vi "Return Transfer Group.vi"(8 "error in (no error)":errorcluster, 10 "Transfer Group in":refnum<class "Transfer Group.lvclass">, 11 "Transceiver Thread in":refnum<class "Plugin Thread.lvclass">) -> (0 "error out":errorcluster, 3 "Transceiver Thread out":refnum<class "Plugin Thread.lvclass">)   [LabVIEW 2017, in "DSF Core.lvlib" / "Plugin Thread.lvclass"]
uses:
  Thread/Plugin/Plugin Thread.lvclass
  Transfer Group/Transfer Group.lvclass
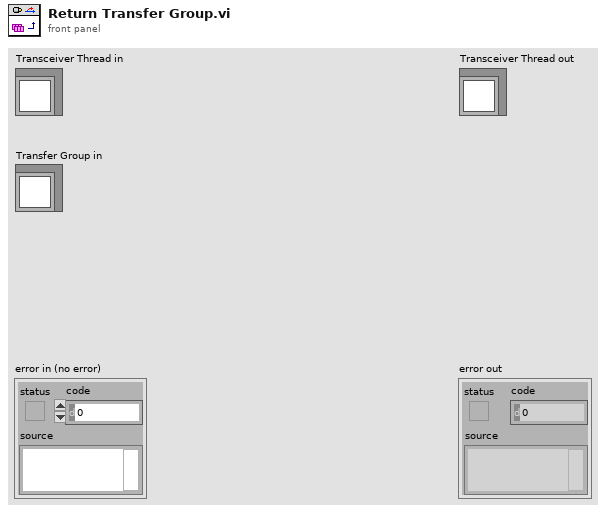
[diagram p1: front panel]
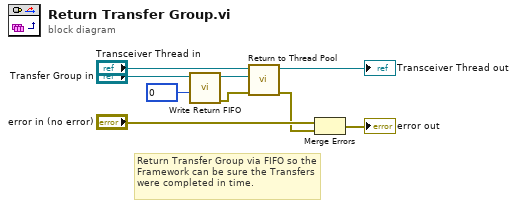
[diagram p0: block diagram]
diagram:
  # "Return Transfer Group via FIFO so the Framework can be sure the Transfers were completed in time."
  n1 = call "Write Return FIFO.vi"("timeout in ms (0)"=0, "Transfer Group in"="Transfer Group in") -> ("error out"=w2:errorcluster, "Transfer Group out"=w4:refnum<class "Transfer Group.lvclass">)  [unwired: 7 in, 1 out]
  n2 = call "Return to Thread Pool.vi"("error in (no error)"=w2, "Transfer Group in"=w4, "Plugin Thread in"="Transceiver Thread in") -> ("error out"=w1:errorcluster, "Plugin Thread out"=→"Transceiver Thread out":refnum<class "Plugin Thread.lvclass">)  [unwired: 7 in]
  n3 = Merge Errors("error in (no error)", w1) -> (→"error out":errorcluster)
